vi "FGV - Module Path.vi"(6 "FGV State":T1=enum."Read", 8 "Error In":errorcluster, 11 "Path In":path) -> (0 "Error Out":errorcluster, 3 "Path Out":path)   [LabVIEW 2020]
doc: "This FGV carry path for system. The path is at same location as exe file."
uses:
  Control/State - FGV.ctl
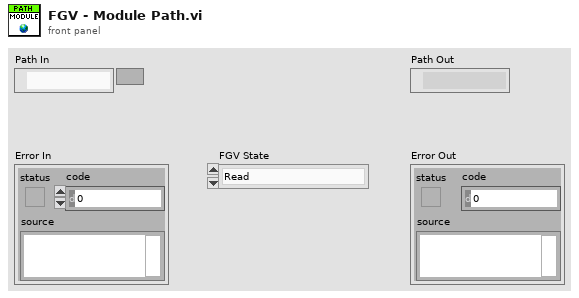
[diagram p1: front panel]
types:
  T1 = typedef "State - FGV.ctl" = enum16{"Write", "Read"}
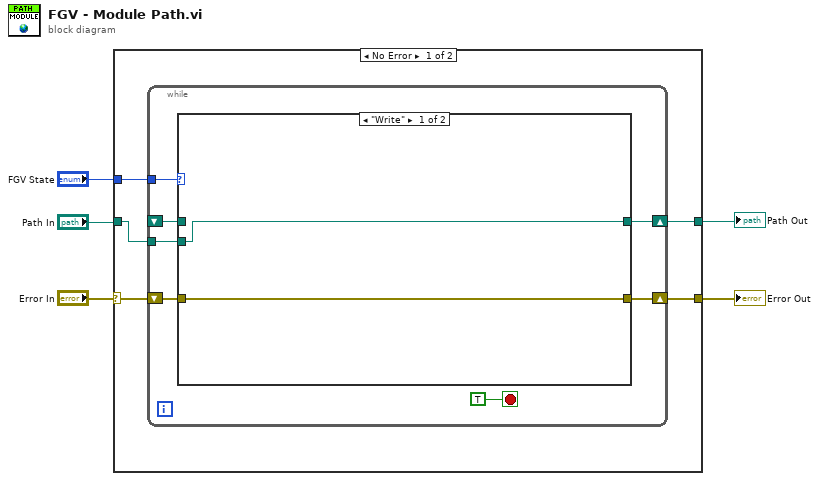
[diagram p0: block diagram]
diagram:
  n1 = case shown="No Error" "Error In" {
    selector: "Error In" -> [w9 w23]
    tunnel: "FGV State" -> [w8 _]
    tunnel: [w10 w23] -> w5
    tunnel: "Path In" -> [w7 w22]
    tunnel: [w6 w22] -> w1
    frame No Error {
      n2 = while {
        tunnel: w8 -> [w14]
        shift-right: [w17] -> w10
        shift-left: w9 -> [w16]
        shift-right: [w12] -> w6
        shift-left: _ -> [w13]
        tunnel: w7 -> [w11]
        stop <- TRUE stop-if-true
        n3 = case shown="\"Write\"" w14 {
          tunnel: w16 -> [w19 w21]
          tunnel: [w19 w21] -> w17
          tunnel: w13 -> [_ w20]
          tunnel: [w18 w20] -> w12
          tunnel: w11 -> [w18 _]
          frame "Write" {
          }
          frame "Read" {
          }
        }
      }
    }
    frame Error {
    }
  }
  "Error Out" <- w5
  "Path Out" <- w1
